vi "Begin.vi"() -> (0 "error out":errorcluster)   [LabVIEW 2015]
doc: "Called before other user functions, this VI is expected to open initial I/O refnums, load in file data, and do all program initialization. Notice that the <B>error out</B> terminal is simply used for data flow. Wiring it to other structures or subVIs ensures that this VI runs first."
uses:
  <vilib>/Rock Robotics/WPI/DriverStation/WPI_DriverStationRobotMode2.ctl
  <vilib>/Rock Robotics/WPI/Joystick/WPI_JoystickDeviceEnum.ctl
  Robot Global Data.vi
  navX-MXP-LabVIEW/navX-MXP Library/navX-MXP IMU.lvlib
  900/Team900-VIs/Team900SwerveDrive/Team900SwerveDrive.lvlib
panel:
  in  "Pivot PID":T1={"No Bin"={"P"=15.0, "I"=0.0, "D"=0.0}, "Bin"={"P"=20.0, "I"=0.0, "D"=0.0}}
  in  "Extension PID":T1={"No Bin"={"P"=19.0, "I"=0.0, "D"=0.0}, "Bin"={"P"=19.0, "I"=0.0, "D"=0.0}}
  in  "Wrist PID":T1={"No Bin"={"P"=20.0, "I"=0.0, "D"=0.0}, "Bin"={"P"=30.0, "I"=0.0, "D"=0.0}}
  in  "Ramp Rate":dbl=50.0
  in  "Speed PID":cluster{"P":dbl, "I":dbl, "D":dbl}={"P"=0.0275, "I"=0.000115, "D"=0.682955}
  in  "Steering PID":cluster{"P":dbl, "I":dbl, "D":dbl}={"P"=48.0, "I"=0.0, "D"=638.0}
  in  "error in":errorcluster
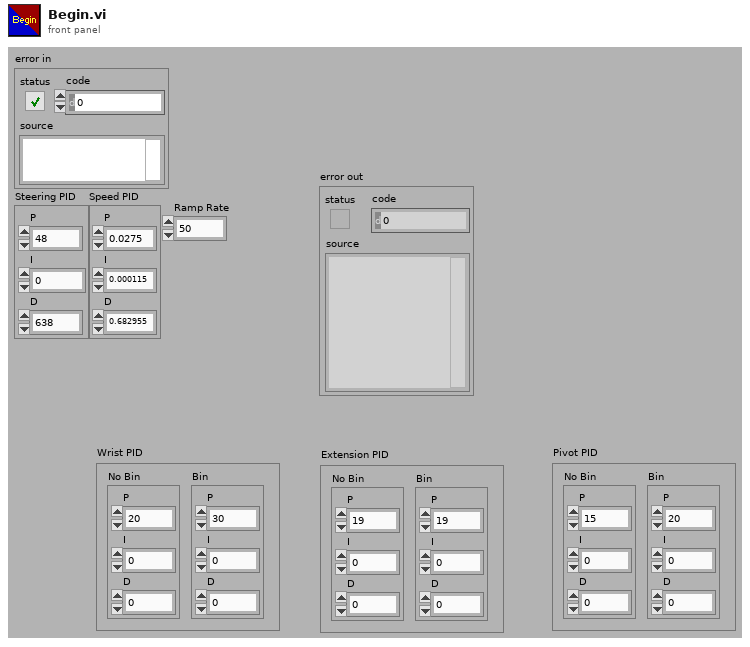
[diagram p1: front panel]
types:
  T1 = cluster{"No Bin":cluster{"P":dbl, "I":dbl, "D":dbl}, "Bin":cluster{"P":dbl, "I":dbl, "D":dbl}}
  T2 = typedef "WPI_DriverStationRobotMode2.ctl" = enum16{"Autonomous Disabled", "Autonomous Enabled", "Teleop Disabled", "Teleop Enabled", "Disconnected", "Finish", "Test Disabled", "Test Enabled", "Emergency Stopped"}
  T3 = typedef "WPI_JoystickDeviceEnum.ctl" = enum16{"USB 0", "USB 1", "USB 2", "USB 3", "USB 4", "USB 5"}
  T4 = typedef "WPI_JoystickDevRef.ctl" = cluster{"Device":T3}
  T5 = typedef "navX-MXP IMU.lvlib/navX Device TypeDef.ctl" = cluster{"navX Interface Protocol":T6, "navX Interface Protocol TypeDefs":cluster{"SPIDevRef":T7, "I2CDevRef":T9}, "navX System Information":cluster{"Board Information":T11, "Status":T12, "Offsets":T16}, "navX Common Information":cluster{"Update Rate (4Hz-60Hz)":T17, "refnum name":string, "error":errorcluster}}
  T6 = typedef "navX-MXP IMU.lvlib/navX Interface Protocol.ctl" = enum16{"SPI", "I2C"}
  T7 = typedef "WPI_SPIDevRef.ctl" = cluster{"DevStatus":errorcluster, "Handle":i32, "SPI Bus":T8}
  T8 = typedef "spi_bus.ctl" = enum16{"SPI On-Board, CS0", "SPI On-Board, CS1", "SPI On-Board, CS2", "SPI On-Board, CS3", "SPI MXP", "Invalid"}
  T9 = typedef "WPI_I2CDevRef.ctl" = cluster{"DevStatus":errorcluster, "Device Address":u8, "Handle":i32, "I2C Bus":T10}
  T10 = typedef "i2c_bus.ctl" = enum16{"I2C On-Board", "I2C MXP", "Invalid"}
  T11 = typedef "navX-MXP IMU.lvlib/navX Board Information.ctl" = cluster{"WhoAmI (50 | 0x32)":u8, "Board Revision":u8, "Firmware Major Version":u8, "Firmware Minor Version":u8}
  T12 = typedef "navX-MXP IMU.lvlib/navX Status Data.ctl" = cluster{"Update Rate Hz":u8, "Accelerometer Full-Scale Range":u8, "Gyro Full-Scale Range":u16, "NAVX_OP_STATUS":T13, "NAVX_CAL_STATUS":T14, "NAVX_SELFTEST_STATUS":u8, "NAVX_SENSOR_STATUS":T15}
  T13 = typedef "navX-MXP IMU.lvlib/navX NAVX_OP_STATUS.ctl" = u8
  T14 = typedef "navX-MXP IMU.lvlib/navX NAVX_CAL_STATUS.ctl" = u8
  T15 = typedef "navX-MXP IMU.lvlib/navX NAVX_SENSOR_STATUS.ctl" = cluster{"MOVING":bool, "YAW_STABLE":bool, "MAG_DISTURBANCE":bool, "ALTITUDE_VALID":bool, "SEALEVEL_PRESS_SET":bool, "FUSED_HEADING_VALID":bool}
  T16 = typedef "navX-MXP IMU.lvlib/navX Offsets Data.ctl" = cluster{"Yaw":dbl, "Quat W":dbl, "Quat X":dbl, "Quat Y":dbl, "Quat Z":dbl}
  T17 = typedef "navX-MXP IMU.lvlib/navX Update Rate.ctl" = u8
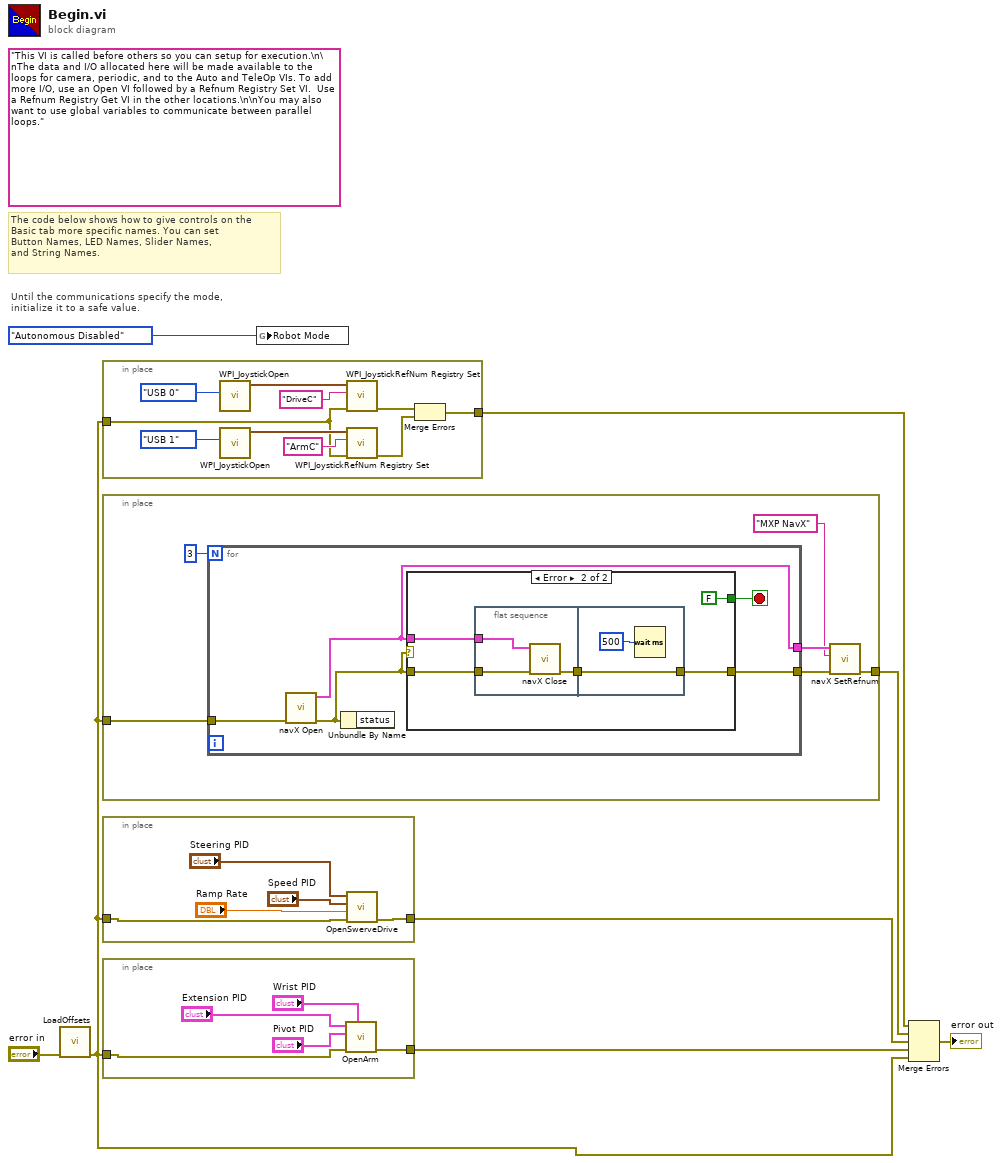
[diagram p0: block diagram]
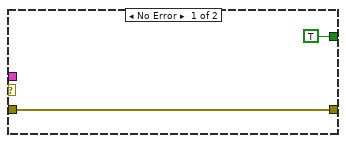
[diagram p2: hidden frame]
diagram:
  (unwired) "This VI is called before others so you can setup for execution.\n\nThe data and I/O allocated here will be made available to the loops for camera, periodic, and to the Auto and TeleOp VIs. To add more I/O, use an Open VI followed by a Refnum Registry Set VI.  Use a Refnum Registry Get VI in the other locations.\n\nYou may also want to use global variables to communicate between parallel loops."
  # "The code below shows how to give controls on the\nBasic tab more specific names. You can set\nButton Names, LED Names, Slider Names,\nand String Names."
  # "Until the communications specify the mode,\ninitialize it to a safe value."
  n1 = call "LoadOffsets.vi"("error in (no error)"="error in") -> ("error out"=w1:errorcluster)  [unwired: 10 in]
  n2 = in-place {
    in-place-border: [w10] -> w6
    in-place-border: w1 -> [w11]
    n3 = call <vilib>:"WPI_JoystickOpen.vi"("JoystickDevice"=WPI_JoystickDeviceEnum."USB 0") -> ("JoystickDevRef"=w17:T4)  [unwired: 10 in]
    n4 = call <vilib>:"WPI_JoystickOpen.vi"("JoystickDevice"=WPI_JoystickDeviceEnum."USB 1") -> ("JoystickDevRef"=w14:T4)  [unwired: 10 in]
    n5 = call <vilib>:"WPI_JoystickRefNum Registry Set.vi"("error in (no error)"=w11, "refnum name"="DriveC", "JoystickDevRef"=w17) -> ("error out"=w18:errorcluster)  [unwired: 7 in, 1 out]
    n6 = call <vilib>:"WPI_JoystickRefNum Registry Set.vi"("error in (no error)"=w11, "refnum name"="ArmC", "JoystickDevRef"=w14) -> ("error out"=w9:errorcluster)  [unwired: 7 in, 1 out]
    n7 = Merge Errors(w18, w9) -> (w10:errorcluster)
  }
  n8 = in-place {
    in-place-border: [w24] -> w5
    in-place-border: w1 -> [w21]
    n9 = for {
      N: 3 -> [_]
      tunnel: [w28] -> w22
      tunnel: w21 -> [w29]
      tunnel: [w27] -> w23
      stop <- w25 stop-if-true
      n10 = call "navX Open.vi"("error in"=w29) -> ("error out"=w26:errorcluster, "navX Device TypeDef"=w28:T5)  [unwired: 8 in, 1 out]
      n11 = Unbundle By Name(w26) -> ()  [unwired: 1 out]
      n12 = case shown="Error" w26 {
        tunnel: w26 -> [w31 w35]
        tunnel: w28 -> [_ w36]
        tunnel: [w31 w34] -> w27
        tunnel: [TRUE FALSE] -> w25
        frame No Error {
        }
        frame Error {
          n13 = flat-sequence {
            tunnel: w36 -> [w39]
            tunnel: w35 -> [w38]
            tunnel: [w37] -> w32
            tunnel: [w41] -> w34
            tunnel: w32 -> [w41]
            frame #0 {
              n14 = call "navX Close.vi"("error in (no error)"=w38, "navX Device TypeDef"=w39) -> ("error out"=w37:errorcluster)  [unwired: 9 in]
            }
            frame #1 {
              n15 = Wait (ms)(milliseconds to wait=u32 500) -> ()  [unwired: 1 out]
            }
          }
        }
      }
    }
    n16 = call "navX SetRefnum.vi"("error in (no error)"=w23, "refnum name"="MXP NavX", "navX Device TypeDef"=w22) -> ("error out"=w24:errorcluster)  [unwired: 7 in, 1 out]
  }
  n17 = in-place {
    in-place-border: [w42] -> w4
    in-place-border: w1 -> [w46]
    n18 = call "OpenSwerveDrive.vi"("error in"=w46, "Ramp Rate"="Ramp Rate", "Speed PID"="Speed PID", "Steering PID"="Steering PID") -> ("error out"=w42:errorcluster)  [unwired: 5 in]
  }
  n19 = in-place {
    in-place-border: [w51] -> w3
    in-place-border: w1 -> [w50]
    n20 = call "OpenArm.vi"("Wrist PID"="Wrist PID", "error in (no error)"=w50, "Pivot PID"="Pivot PID", "Extension PID"="Extension PID") -> ("error out"=w51:errorcluster)  [unwired: 7 in]
  }
  n21 = global write "Robot Global Data.vi" "Robot Mode"(WPI_DriverStationRobotMode2."Autonomous Disabled" ("Robot Mode")) -> ()
  n22 = Merge Errors(w6, w5, w4, w3, w1) -> (→"error out":errorcluster)
